vi "Build dotNET Custom Actions.vi"(8 "error in (no error)":errorcluster, 11 "Bundle Builder in":refnum<class "Bundle Builder.lvclass">) -> (0 "error out":errorcluster, 2 "Custom Actions":refnum<k24>[](array[refnum]), 3 "Bundle Builder out":refnum<class "Bundle Builder.lvclass">)   [LabVIEW 2020, in "Bundle Builder.lvclass"]
uses:
  Bundle Builder.lvclass
  C:/Users/chihong/Documents/Repos/StsCustomBundleBuilder/Code/StsCustomBundleBuilder/StsCustomBundleBuilderLib/StsCustomBundleBuilderLib.dll
  StsCustomBundleBuilderLib/StsCustomBundleBuilderLib.dll
  Bundle Builder.lvclass/Bundle Builder.ctl
  <vilib>/Utility/error.llb/Error Cluster From Error Code.vi
  <vilib>/ErrorRing/Error Ring.xnode
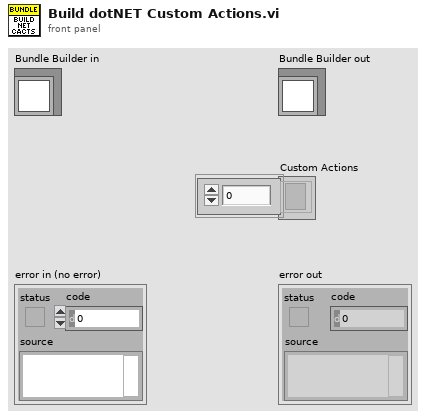
[diagram p1: front panel]
types:
  T1 = cluster{"Display Name":string, "Commands":cluster{"Path":string, "Parameters":string, "Successful Exit Codes":string}[]}[]
  T2 = cluster{"Path":string, "Parameters":string, "Successful Exit Codes":string}[]
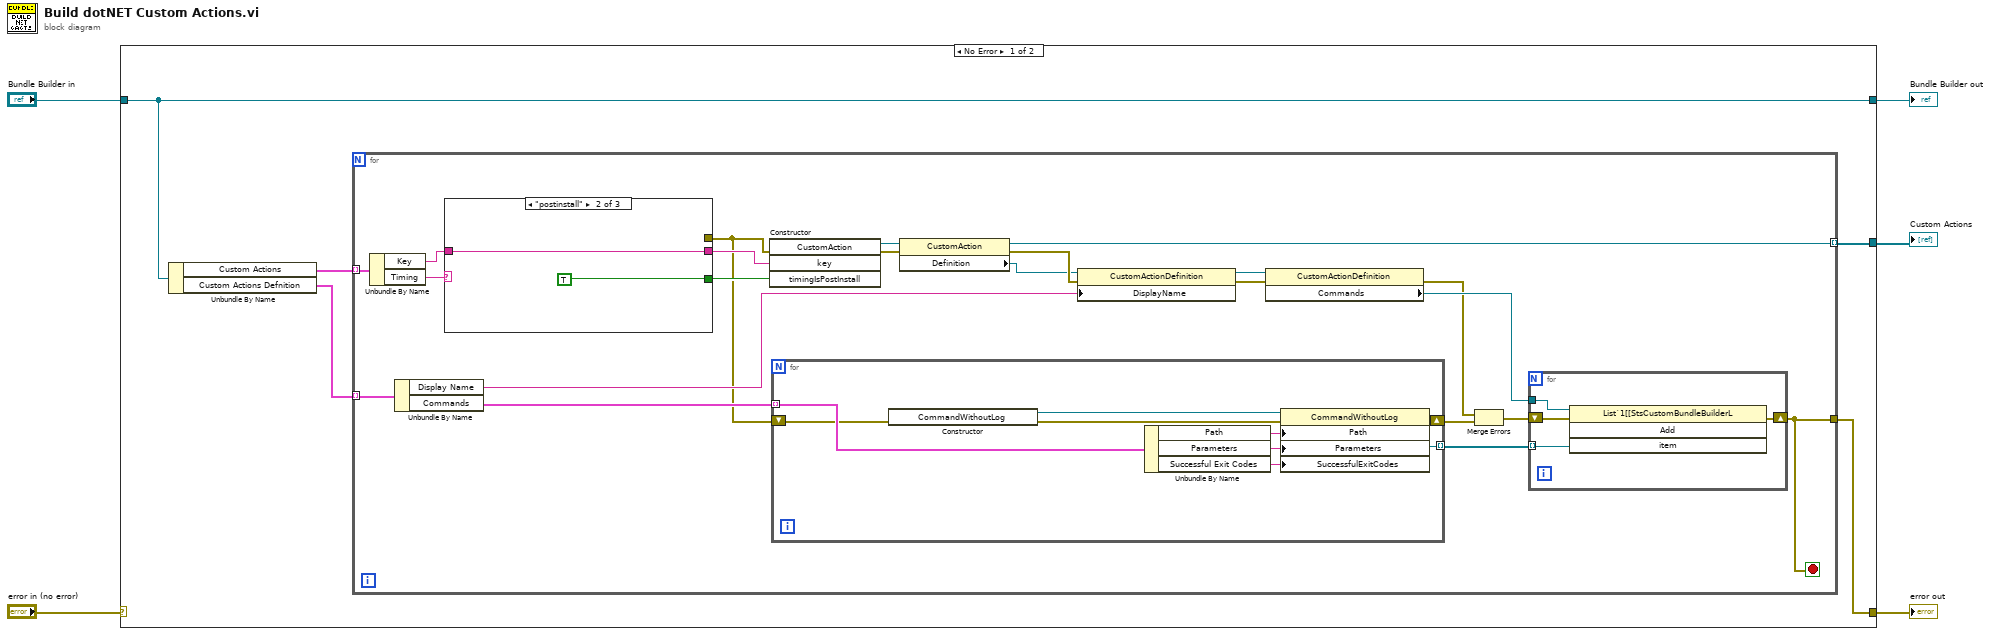
[diagram p0: block diagram]
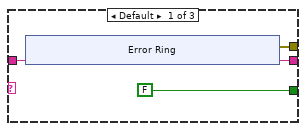
[diagram p2: hidden frame]
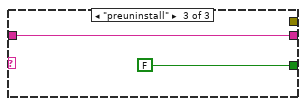
[diagram p3: hidden frame]
diagram:
  n1 = case shown="No Error" "error in (no error)" {
    selector: "error in (no error)" -> [_ w61]
    tunnel: [w7 w61] -> w4
    tunnel: [w8 w60] -> w2
    tunnel: "Bundle Builder in" -> [w8 w60]
    tunnel: [w6 _] -> w1
    frame No Error {
      n2 = Unbundle By Name(w8) -> ("Custom Actions"=w10:cluster{"Key":string, "Timing":string}[], "Custom Actions Defnition"=w9:T1)
      n3 = for {
        tunnel: w10 -> [w30] mode=indexing
        tunnel: w9 -> [w32] mode=indexing
        tunnel: [w23] -> w7
        tunnel: [w11] -> w6 mode=indexing
        stop <- w23 stop-if-true
        n4 = Unbundle By Name(w30) -> ("Key"=w14:string, "Timing"=w16:string)
        n5 = Unbundle By Name(w32) -> ("Display Name"=w29:string, "Commands"=w31:T2)
        n6 = case shown="\"postinstall\"" w16 {
          tunnel: [FALSE TRUE FALSE] -> w15
          tunnel: w14 -> [w47 w56 w58]
          tunnel: [w47 w56 w58] -> w13
          tunnel: [w46 _ _] -> w12
          frame Default {
            n7 = xnode "Error Ring"("parameter 0"=w47) -> ("error out"=w46:errorcluster)
          }
          frame "postinstall" {
          }
          frame "preuninstall" {
          }
        }
        n8 = constructor class="CustomAction"(error in=w12, "key"=w13, "timingIsPostInstall"=w15) -> (reference out=w18:refnum<k24>, error out=w22:errorcluster)  [unwired: 2 in, 3 out]
        n9 = for {
          tunnel: w31 -> [w40] mode=indexing
          tunnel: [w36] -> w25 mode=indexing
          shift-right: [w34] -> w27
          shift-left: w12 -> [w33]
          n10 = constructor class="CommandWithoutLog"(error in=w33) -> (reference out=w41:refnum<k24>, error out=w35:errorcluster)  [unwired: 2 in, 1 out]
          n11 = Unbundle By Name(w40) -> ("Path"=w39:string, "Parameters"=w38:string, "Successful Exit Codes"=w37:string)
          n12 = property class="CommandWithoutLog"(reference=w41, error in=w35, "Path"=w39, "Parameters"=w38, "SuccessfulExitCodes"=w37) -> (reference out=w36:refnum<k24>, error out=w34:errorcluster)
        }
        n13 = property class="CustomAction"(reference=w18, error in=w22) -> (reference out=w11:refnum<k24>, error out=w19:errorcluster, "Definition"=w17:refnum<k24>)
        n14 = property class="CustomActionDefinition"(reference=w17, error in=w19, "DisplayName"=w29) -> (reference out=w21:refnum<k24>, error out=w20:errorcluster)
        n15 = property class="CustomActionDefinition"(reference=w21, error in=w20) -> (error out=w24:errorcluster, "Commands"=w28:refnum<k24>)  [unwired: 1 out]
        n16 = Merge Errors(w24, w27) -> (w26:errorcluster)
        n17 = for {
          tunnel: w28 -> [w42]
          shift-right: [w43] -> w23
          shift-left: w26 -> [w45]
          tunnel: w25 -> [w44] mode=indexing
          n18 = invoke class="List`1[[StsCustomBundleBuilderL" method="Add"(reference=w42, error in=w45, "item"=w44) -> (error out=w43:errorcluster)  [unwired: 1 in, 3 out]
        }
      }
    }
    frame Error {
    }
  }
  "error out" <- w4
  "Bundle Builder out" <- w2
  "Custom Actions" <- w1
